vi "ReadRampInfo.vi"(8 "error in (no error)":errorcluster, 11 "VISA Refnum in":refnum<visa-resource-name>) -> (0 "error in (no error) 2":errorcluster, 1 "Cooling Ramp °C/s":dbl, 2 "Heating Ramp °C/s":dbl, 3 "VISA Refnum Out":refnum<visa-resource-name>, 5 "Time base (s)":dbl)   [LabVIEW 2023]
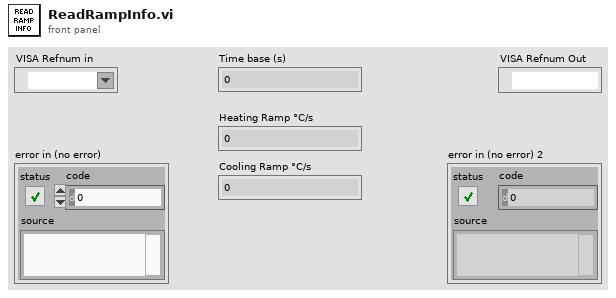
[diagram p1: front panel]
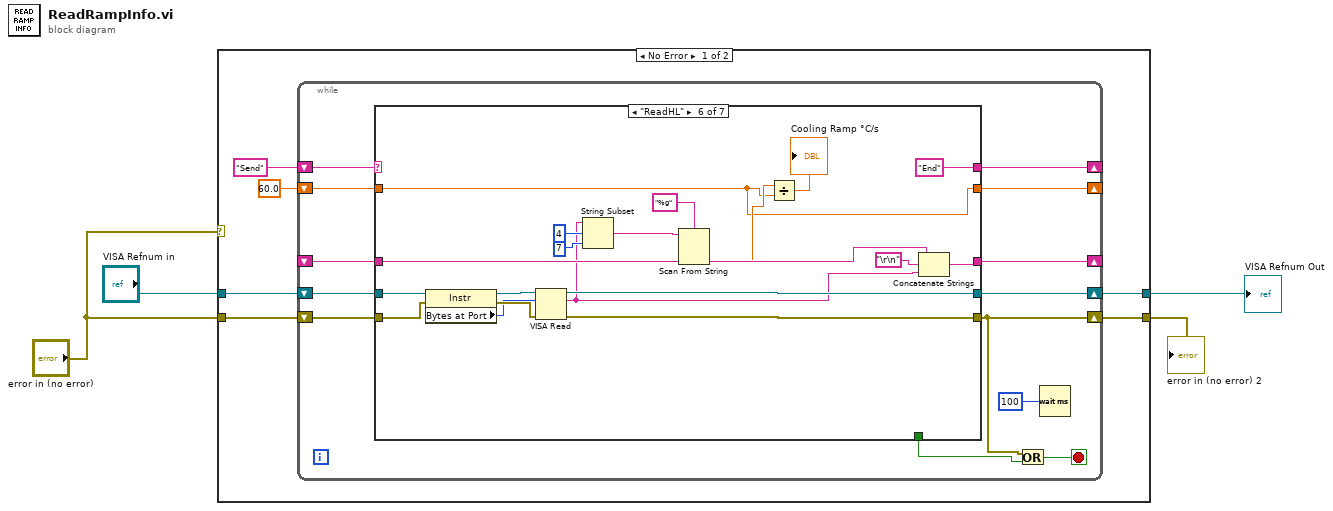
[diagram p0: block diagram]
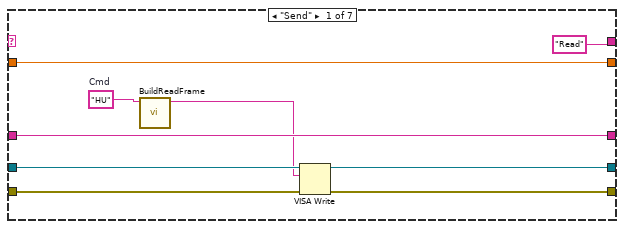
[diagram p2: hidden frame]
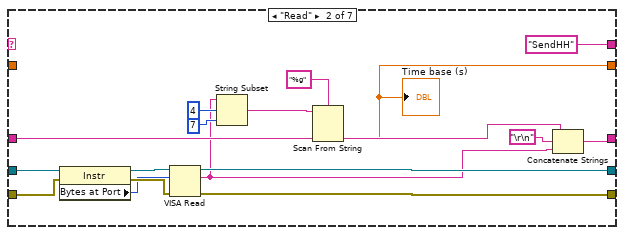
[diagram p3: hidden frame]
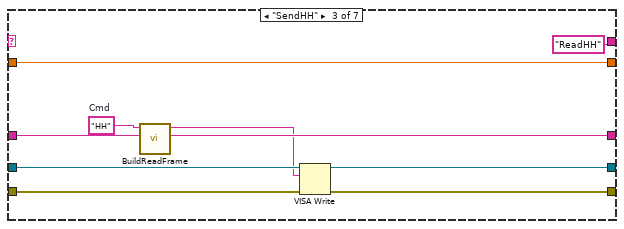
[diagram p4: hidden frame]
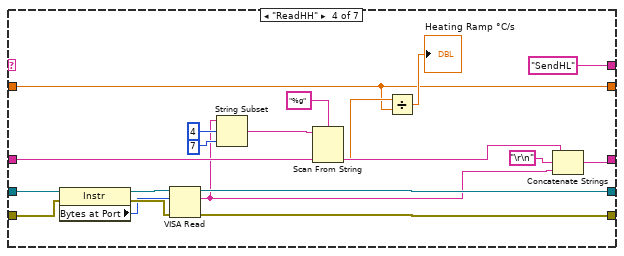
[diagram p5: hidden frame]
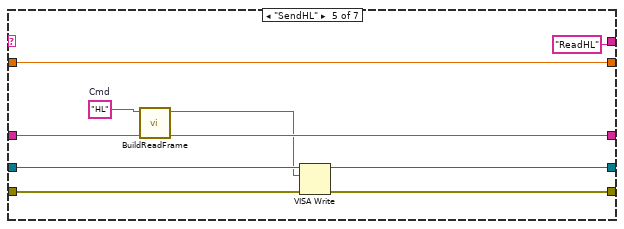
[diagram p6: hidden frame]
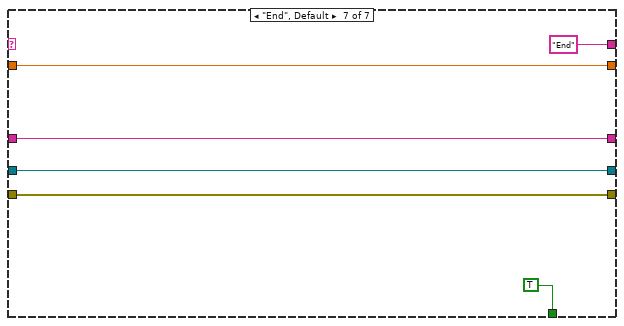
[diagram p7: hidden frame]
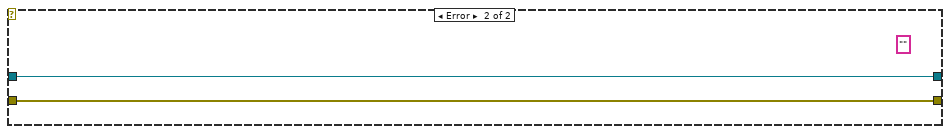
[diagram p8: hidden frame]
diagram:
  n1 = case shown="No Error" "error in (no error)" {
    tunnel: "VISA Refnum in" -> [w10 w113]
    tunnel: "error in (no error)" -> [w9 w112]
    tunnel: [w7 w113] -> w1
    tunnel: [w6 w112] -> w2
    frame No Error {
      n2 = while {
        shift-right: [w20] -> _
        shift-left: "Send" -> [w21]
        shift-right: [w15] -> w7
        shift-left: w10 -> [w23]
        shift-right: [w16] -> w6
        shift-left: w9 -> [w22]
        shift-right: [w14] -> _
        shift-left: _ -> [w13]
        shift-right: [w12] -> _
        shift-left: 60.0 ("Time base (s)") -> [w11]
        stop <- w18 stop-if-true
        n3 = case shown="\"ReadHL\"" w21 {
          tunnel: w23 -> [w31 w49 w57 w77 w85 w105 w109]
          tunnel: w22 -> [w30 w48 w56 w76 w84 w104 w110]
          tunnel: ["Read" "SendHH" "ReadHH" "SendHL" "ReadHL" "End" "End"] -> w20
          tunnel: [_ _ _ _ _ _ TRUE] -> w17
          tunnel: [w28 w43 w54 w71 w82 w99 w110] -> w16
          tunnel: [w27 w44 w53 w72 w81 w100 w109] -> w15
          tunnel: [w26 w34 w52 w62 w80 w90 w107] -> w14
          tunnel: w13 -> [w26 w36 w52 w64 w80 w92 w107]
          tunnel: [w24 w33 w50 w59 w78 w87 w106] -> w12
          tunnel: w11 -> [w24 _ w50 w59 w78 w87 w106]
          frame "Send" {
            w32 = "HU"  # Cmd
            n4 = call "BuildReadFrame.vi"("Cmd"=w32) -> ("String"=w25:string)  [unwired: 10 in]
            n5 = VISA Write(VISA resource name=w31, write buffer=w25, error in (no error)=w30) -> (VISA resource name out=w27:refnum<visa-resource-name>, error out=w28:errorcluster)  [unwired: 1 out]
          }
          frame "Read" {
            n6 = property class="Instr"(reference=w49, error in=w48) -> (reference out=w47:refnum<visa-resource-name>, error out=w46:errorcluster, "Bytes at Port"=w45:u32)
            n7 = VISA Read(VISA resource name=w47, byte count=w45, error in (no error)=w46) -> (VISA resource name out=w44:refnum<visa-resource-name>, read buffer=w35:string, error out=w43:errorcluster)  [unwired: 1 out]
            n8 = String Subset(string=w35, offset (0)=4, length (rest)=7 ("length (rest)")) -> (substring=w38:string)
            n9 = Scan From String(format string="%g", input string=w38) -> (output 1=w33:dbl)  [unwired: 3 in, 3 out]
            "Time base (s)" <- w33
            n10 = Concatenate Strings(w36, "\r\n", w35) -> (w34:string)
          }
          frame "SendHH" {
            w58 = "HH"  # Cmd
            n11 = call "BuildReadFrame.vi"("Cmd"=w58) -> ("String"=w51:string)  [unwired: 10 in]
            n12 = VISA Write(VISA resource name=w57, write buffer=w51, error in (no error)=w56) -> (VISA resource name out=w53:refnum<visa-resource-name>, error out=w54:errorcluster)  [unwired: 1 out]
          }
          frame "ReadHH" {
            n13 = property class="Instr"(reference=w77, error in=w76) -> (reference out=w75:refnum<visa-resource-name>, error out=w74:errorcluster, "Bytes at Port"=w73:u32)
            n14 = VISA Read(VISA resource name=w75, byte count=w73, error in (no error)=w74) -> (VISA resource name out=w72:refnum<visa-resource-name>, read buffer=w63:string, error out=w71:errorcluster)  [unwired: 1 out]
            n15 = String Subset(string=w63, offset (0)=4, length (rest)=7 ("length (rest)")) -> (substring=w66:string)
            n16 = Scan From String(format string="%g", input string=w66) -> (output 1=w60:dbl)  [unwired: 3 in, 3 out]
            n17 = Divide(x=w60, y=w59) -> (x/y=→"Heating Ramp °C/s":dbl)
            n18 = Concatenate Strings(w64, "\r\n", w63) -> (w62:string)
          }
          frame "SendHL" {
            w86 = "HL"  # Cmd
            n19 = call "BuildReadFrame.vi"("Cmd"=w86) -> ("String"=w79:string)  [unwired: 10 in]
            n20 = VISA Write(VISA resource name=w85, write buffer=w79, error in (no error)=w84) -> (VISA resource name out=w81:refnum<visa-resource-name>, error out=w82:errorcluster)  [unwired: 1 out]
          }
          frame "ReadHL" {
            n21 = property class="Instr"(reference=w105, error in=w104) -> (reference out=w103:refnum<visa-resource-name>, error out=w102:errorcluster, "Bytes at Port"=w101:u32)
            n22 = VISA Read(VISA resource name=w103, byte count=w101, error in (no error)=w102) -> (VISA resource name out=w100:refnum<visa-resource-name>, read buffer=w91:string, error out=w99:errorcluster)  [unwired: 1 out]
            n23 = String Subset(string=w91, offset (0)=4, length (rest)=7 ("length (rest)")) -> (substring=w94:string)
            n24 = Scan From String(format string="%g", input string=w94) -> (output 1=w88:dbl)  [unwired: 3 in, 3 out]
            n25 = Divide(x=w88, y=w87) -> (x/y=→"Cooling Ramp °C/s":dbl)
            n26 = Concatenate Strings(w92, "\r\n", w91) -> (w90:string)
          }
          frame "End", Default {
          }
        }
        n27 = Or(x=w16, y=w17) -> (x .or. y?=w18:bool)
        n28 = Wait (ms)(milliseconds to wait=u32 100) -> ()  [unwired: 1 out]
      }
    }
    frame Error {
      (unwired) "" ("read buffer")
    }
  }
  "VISA Refnum Out" <- w1
  "error in (no error) 2" <- w2
